vi "986x.Create.vi"(8 "error in (no error)":errorcluster, 10 "986x Support":T2, 11 "Device Item Ref in":T1 format="%.0x") -> (0 "error out":errorcluster, 3 "Device Ref out":T1 format="%.0x")   [LabVIEW 2019, in "Ghost Bus Addon System Explorer.lvlib"]
uses:
  Ghost Bus Addon System Explorer.lvlib
  <vilib>/NI VeriStand/Custom Device API/Custom Device Item Ref.ctl
  Addon Shared/Types/986x.ctl
  Addon Shared/SubVIs/GUID Lookup.vi
  <vilib>/NI/NI VeriStand Advanced SysDef API/_SubVIs/SysDef.Property.Set.Boolean.vi
  <vilib>/NI/NI VeriStand Advanced SysDef API/_SubVIs/SysDef.Property.Set.String.vi
  <vilib>/Utility/MD5Checksum.llb/MD5Checksum File.vi
  <vilib>/NI/NI VeriStand Advanced SysDef API/_SubVIs/SysDef.Property.Set.DependentFile.vi
  <vilib>/NI/NI VeriStand Advanced SysDef API/SysDef API/SysDef.Property.Remove.vi
  <vilib>/NI/NI VeriStand Advanced SysDef API/SysDef API/Advanced System Definition.lvlib
  Addon Shared/Ghost Bus Addon Shared.lvlib
  <vilib>/NI VeriStand/Custom Device API/Custom Device API.lvlib
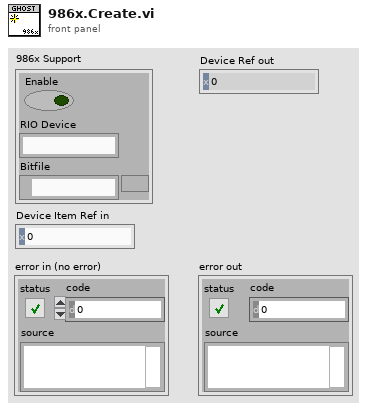
[diagram p1: front panel]
types:
  T1 = typedef "Custom Device API.lvlib/Custom Device Item Ref.ctl" = u64
  T2 = typedef "Ghost Bus Addon Shared.lvlib/986x.ctl" = cluster{"Enable":bool, "RIO Device":string, "Bitfile":path}
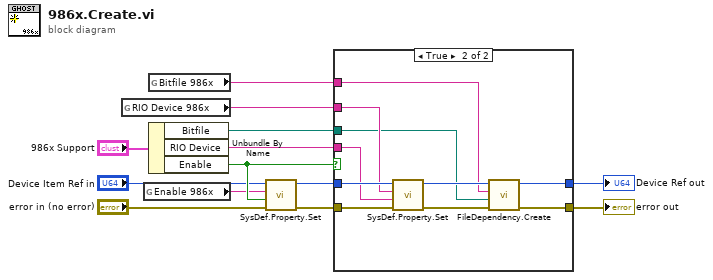
[diagram p0: block diagram]
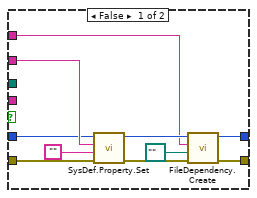
[diagram p2: hidden frame]
diagram:
  n1 = global read "GUID Lookup.vi" "RIO Device 986x"() -> (w2:string)
  n2 = global read "GUID Lookup.vi" "Enable 986x"() -> (w1:string)
  n3 = global read "GUID Lookup.vi" "Bitfile 986x"() -> (w3:string)
  n4 = Unbundle By Name("986x Support") -> ("Bitfile"=w13:path, "RIO Device"=w12:string, "Enable"=w11:bool)
  n5 = call-poly <vilib>:"SysDef.Property.Set.vi"("error in (no error)"="error in (no error)", "Value"=w11, "Property Name"=w1, "nodeID"="Device Item Ref in") -> ("error out"=w7:errorcluster, "nodeID out"=w9:u64)  [unwired: 6 in]
  n6 = case shown="True" w11 {
    tunnel: w7 -> [w22 w33]
    tunnel: [w19 w28] -> w8
    tunnel: w9 -> [w21 w32]
    tunnel: w2 -> [w23 w30]
    tunnel: [w18 w26] -> w10
    tunnel: w12 -> [_ w31]
    tunnel: w13 -> [_ w25]
    tunnel: w3 -> [w15 w24]
    frame False {
      n7 = call-poly <vilib>:"SysDef.Property.Set.vi"("error in (no error)"=w22, "Value"="", "Property Name"=w23, "nodeID"=w21) -> ("error out"=w20:errorcluster, "nodeID out"=w17:u64)  [unwired: 6 in]
      n8 = call "FileDependency.Create.vi"("error in (no error)"=w20, "DLL Path"=path "" ("Value"), "DLL Property Name"=w15, "Item Ref in"=w17) -> ("error out"=w19:errorcluster, "Item Ref out"=w18:T1)  [unwired: 6 in]
    }
    frame True {
      n9 = call-poly <vilib>:"SysDef.Property.Set.vi"("error in (no error)"=w33, "Value"=w31, "Property Name"=w30, "nodeID"=w32) -> ("error out"=w29:errorcluster, "nodeID out"=w27:u64)  [unwired: 6 in]
      n10 = call "FileDependency.Create.vi"("error in (no error)"=w29, "DLL Path"=w25, "DLL Property Name"=w24, "Item Ref in"=w27) -> ("error out"=w28:errorcluster, "Item Ref out"=w26:T1)  [unwired: 6 in]
    }
  }
  "Device Ref out" <- w10
  "error out" <- w8
